vi "Single Calculate Function.vi"(6 "Source2":i32(ring) caption="Source 2" items=["Input Channel 1", "Input Channel 2", "Input Channel 3", "Input Channel 4", "Calc Channel 1", "Calc Channel 2", "Calc Channel 3", "Calc Channel 4", "Ref Channel 1", "Ref Channel 2", "Ref Channel 3", "Ref Channel 4"], 7 "Operation":i32(ring) items=["Add", "Absolute Value", "Copy", "Derivative", "Integrate", "Invert", "Multiply", "Subtract", "Limit Test", "FFT", "Smooth", "Measurement", "Histogram", "No Operation"], 8 "error in":errorcluster, 9 "Source1":i32(ring) caption="Source 1" items=["Input Channel 1", "Input Channel 2", "Input Channel 3", "Input Channel 4", "Calc Channel 1", "Calc Channel 2", "Calc Channel 3", "Calc Channel 4", "Ref Channel 1", "Ref Channel 2", "Ref Channel 3", "Ref Channel 4"], 10 "Calculation Channel":i32(ring) items=["Calc Channel 1", "Calc Channel 2", "Calc Channel 3", "Calc Channel 4"], 11 "Instrument Handle In":i32) -> (0 "error out":errorcluster, 3 "Instrument Handle Out":i32)   [LabVIEW 8.6, in "ZTScopeM.lvlib"]
doc: "Set a calculation channel to perform an operation."
uses:
  ZTScopeM.lvlib
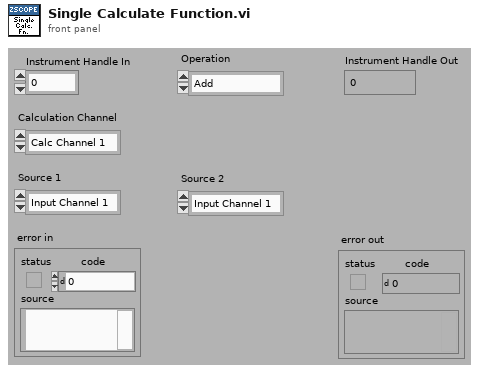
[diagram p1: front panel]
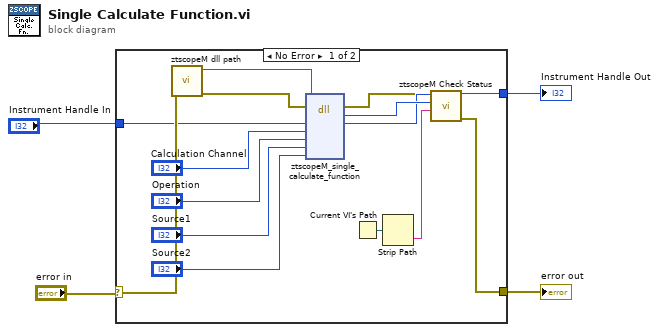
[diagram p0: block diagram]
diagram:
  n1 = case shown="No Error" "error in" {
    selector: "error in" -> [w9 w21]
    tunnel: [w14 w21] -> w3
    tunnel: [w15 w20] -> w2
    tunnel: "Instrument Handle In" -> [w5 w20]
    frame #0 {
      n2 = call "ztscopeM dll path.vi"("error in (no error)"=w9) -> ("error out"=w7:errorcluster, "<instrument>.dll path"=w8:path)  [unwired: 9 in]
      n3 = dll-call lib="C:/Program Files (x86)/National Instruments/LabVIEW 2013/instr.lib/ztscopem/ztscopeM.dll" fn="ztscopeM_single_calculate_function"(path in=w8, error in=w7, "instrumentHandle"=w5, "calculationChannel"="Calculation Channel", "operation"="Operation", "source1"="Source1", "source2"="Source2") -> (error out=w6:errorcluster, w19:i32, "instrumentHandle"=w18:i32)  [unwired: 5 in, 1 out]
      n4 = Current VI's Path() -> (path=w17:path)
      n5 = Strip Path(path=w17) -> (name=w16:string)  [unwired: 1 out]
      n6 = call "ztscopeM Check Status.vi"("error in"=w6, "name of VI"=w16, "status (return code)"=w19, "instrument handle in"=w18) -> ("error out"=w14:errorcluster, "instrument handle out"=w15:i32)  [unwired: 2 out]
    }
    frame #1 {
    }
  }
  "Instrument Handle Out" <- w2
  "error out" <- w3
